vi "CSGaussmeter.setRange.vi"(0 "i ref in":refnum<vi>, 7 "Range":T1, 11 "error in (no error)":errorcluster) -> (4 "i ref out":refnum<vi>, 15 "error out":errorcluster)   [LabVIEW 2014, in "CSGaussmeter.lvlib"]
doc: "This VI sets the Range on 1, 2, 3, 4, 5, 6, 7.\n\n1 = 30 mikro Tesla, 2 = 300 mikro Tesla, 3 = 3 mili Tesla, 4 = 30 mili Tesla, 5 = 300 mili Tesla, 6 = 3 Tesla, 7 = 30 Telar. \n\nDurch das VI kann der Messbereich manuell gewählt werden. Welche Messbereiche vorhanden sind, hängt von der Sonde ab, so dass einige Bereiche eine Fehlermeldung erzeugen können."
uses:
  CSGaussmeter.lvlib
  instr.lib/FH_55/TypeDef/Range.ctl
  CS_Core/CSObj/CSObj.lvlib
  CSlibraries/UtilityLib/UtilityLib.lvlib
  instr.lib/FH_55/FH 55.lvlib
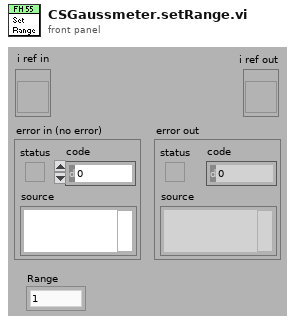
[diagram p1: front panel]
types:
  T1 = typedef "FH 55.lvlib/Range.ctl" = enum16{"1", "2", "3", "4", "5", "6", "7"}
  T2 = typedef "CSGaussmeter.lvlib/CSGaussmeter.i attribute.ctl" = cluster{"Name":string, "VISA Resource Name":refnum<visa-resource-name>, "actValues":cluster{" Limit":bool, "Unit ":T3, "Temp_Unit":T4, "Max":T5, " Filter":bool, " Peak":bool, " Auto_Range":bool, "Range":T1, " Rel":bool, " CTemp":bool, " CField":bool, "AC_DC ":bool, "Set_lower":cluster{"Numeric":dbl, "Cancel Button":bool, "Unit":T6}, "Set_upper":cluster{"Numeric":dbl, "Cancel Button":bool, "Unit":T6}, "Set_Rel":cluster{"Numeric":dbl, "Cancel Button":bool, "Unit":T6}, "Zero":bool, " Local":bool, "Reset":bool, " Init":bool}, "FH 55 Gauss-/Teslameter":T7, "MAX_Value":T8, "MIN_Value":T8, "Rel_Value":T8, "Array ":string[], "LIMU":dbl, " LIML":dbl, "Messwerte 2":string, "Messwerte ":cluster{"Numeric":i32, "OK Button":bool}, "serviceID":cluster{"Current ID":i32, "Unit ID":i32, "Temp ID":i32, "Name ID \n":i32, "Visa ID ":i32}, "setValues ":cluster{" Limit":bool, "Unit ":T3, "Temp_Unit":T4, "Max":T5, " Filter":bool, " Peak":bool, " Auto_Range":bool, "Range":T1, " Rel":bool, " CTemp":bool, " CField":bool, "AC_DC ":bool, "Set_lower":cluster{"Numeric":dbl, "Cancel Button":bool, "Unit":T6}, "Set_upper":cluster{"Numeric":dbl, "Cancel Button":bool, "Unit":T6}, "Set_Rel":cluster{"Numeric":dbl, "Cancel Button":bool, "Unit":T6}, "Zero":bool, " Local":bool, "Reset":bool, " Init":bool}}
  T3 = typedef "FH 55.lvlib/Unit.ctl" = enum16{"T", "G", "A/m"}
  T4 = typedef "FH 55.lvlib/Temp_Unit.ctl" = enum16{"Temp off", "Celsius", "Fahrenheit"}
  T5 = typedef "FH 55.lvlib/Max.ctl" = enum16{"MAX off", "Show MAX", "MAX/MIN"}
  T6 = typedef "FH 55.lvlib/Unit2.ctl" = enum16{"mT", "G", "kA/m"}
  T7 = typedef "FH 55.lvlib/Display.ctl" = cluster{"current value":string, "Limit":string, "Remote":string, "function ":string, "Cluster":cluster{"AC/DC":string, "Auto":string, "Filter":string, "Range":string, "Rel":string, "Peak":string}}
  T8 = typedef "FH 55.lvlib/Value_String.ctl" = cluster{"Numeric":dbl, "String":string}
  T9 = cluster{"VISA Resource Name":refnum<visa-resource-name>}
  T10 = typedef "FH 55.lvlib/VisaCluster.ctl" = cluster{"VISA Resource Name":refnum<visa-resource-name>}
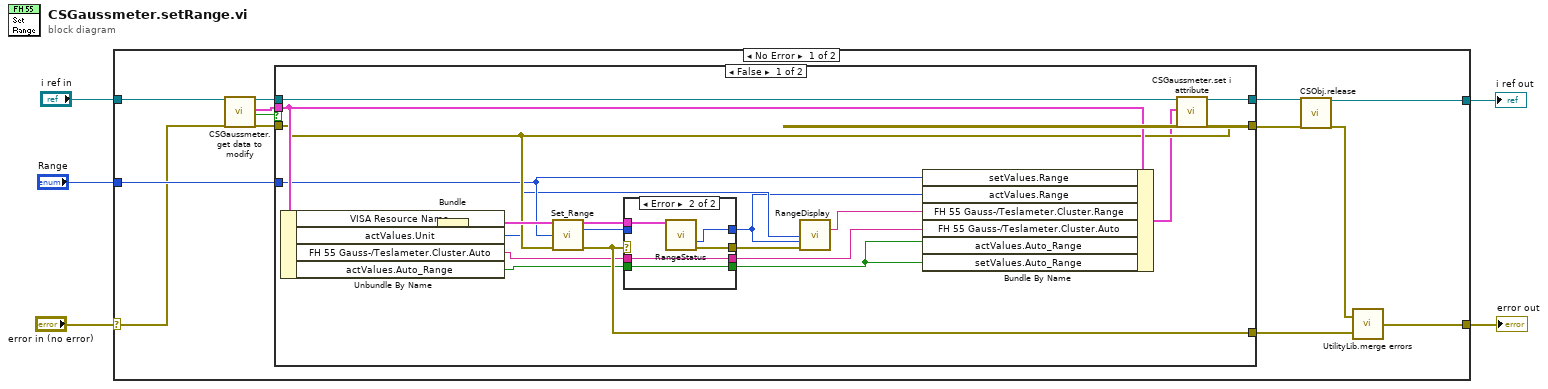
[diagram p0: block diagram]
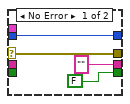
[diagram p2: hidden frame]
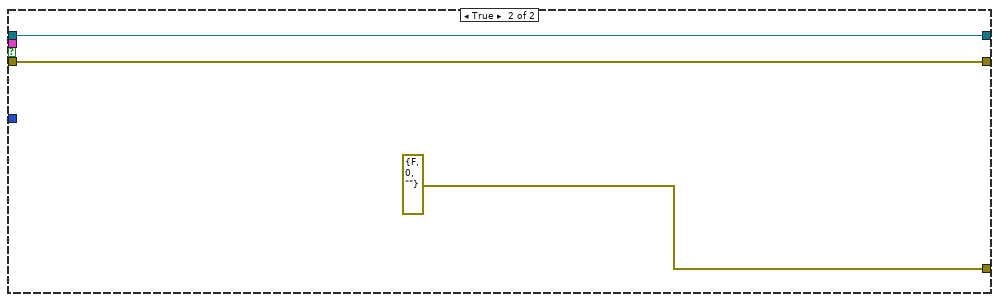
[diagram p3: hidden frame]
diagram:
  n1 = case shown="No Error" "error in (no error)" {
    selector: "error in (no error)" -> [w12 w50]
    tunnel: [w13 w50] -> w2
    tunnel: "i ref in" -> [w11 w51]
    tunnel: [w6 w51] -> w3
    tunnel: "Range" -> [w15 _]
    frame No Error {
      n2 = call "CSGaussmeter.get data to modify.vi"("i ref in"=w11, "error in (no error)"=w12) -> ("i ref out"=w10:refnum<vi>, "i attribute"=w9:T2, "timed out"=w8:bool, "error out"=w7:errorcluster)  [unwired: 14 in]
      n3 = case shown="False" w8 {
        tunnel: w10 -> [w33 w48]
        tunnel: w7 -> [w34 w49]
        tunnel: w9 -> [w36 _]
        tunnel: [w34 w49] -> w16
        tunnel: [w31 w48] -> w18
        tunnel: w15 -> [w30 _]
        tunnel: [w24 errorcluster {"status"=FALSE, "code"=0, "source"=""} ("error out")] -> w14
        frame False {
          n4 = Unbundle By Name(w36) -> ("VISA Resource Name"=w37:refnum<visa-resource-name>, "actValues.Unit"=w29:T3, "FH 55 Gauss-/Teslameter.Cluster.Auto"=w22:string, "actValues.Auto_Range"=w21:bool)
          n5 = Bundle("VISA Resource Name"=w37) -> (w35:T9)  [unwired: 1 in]
          n6 = call "Set_Range.vi"("VisaCluster"=w35, "Range"=w30, "error in (no error)"=w34) -> ("VisaCluster"=w26:T10, "Range"=w28:T1, "error out"=w24:errorcluster)  [unwired: 9 in, 1 out]
          n7 = case shown="Error" w24 {
            selector: w24 -> [w40 _]
            tunnel: w28 -> [w41 _]
            tunnel: [w41 w46] -> w27
            tunnel: w26 -> [_ w45]
            tunnel: [w40 w44] -> w25
            tunnel: w22 -> [_ w42]
            tunnel: w21 -> [_ w43]
            tunnel: ["" w42] -> w20
            tunnel: [FALSE w43] -> w19
            frame No Error {
            }
            frame Error {
              n8 = call "RangeStatus.vi"("VisaCluster"=w45) -> ("Range"=w46:T1, "error out"=w44:errorcluster)  [unwired: 11 in, 2 out]
            }
          }
          n9 = call "RangeDisplay.vi"("Unit"=w29, "Range"=w27, "error in (no error)"=w25) -> ("Display"=w23:string)  [unwired: 10 in, 2 out]
          n10 = Bundle By Name(cluster=w36, "setValues.Range"=w30, "actValues.Range"=w27, "FH 55 Gauss-/Teslameter.Cluster.Range"=w23, "FH 55 Gauss-/Teslameter.Cluster.Auto"=w20, "actValues.Auto_Range"=w19, "setValues.Auto_Range"=w19) -> (w32:T2)
          n11 = call "CSGaussmeter.set i attribute.vi"("i ref in"=w33, "i attribute"=w32) -> ("i ref out"=w31:refnum<vi>)  [unwired: 16 in, 1 out]
        }
        frame True {
        }
      }
      n12 = call "CSObj.release.vi"("i ref in"=w18, "error in (no error)"=w16) -> ("i ref out"=w6:refnum<vi>, "error out"=w17:errorcluster)  [unwired: 16 in]
      n13 = call "UtilityLib.merge errors.vi"("error2 (no error)"=w14, "error1 (no error)"=w17) -> ("error out"=w13:errorcluster)
    }
    frame Error {
    }
  }
  "i ref out" <- w3
  "error out" <- w2
